vi "Add Property to Schema.vi"(4 "Typedef Name":string, 6 "Typedef?":bool, 8 "error in":errorcluster, 9 "JSON Schema Property in":string, 10 "Property Name":string, 11 "JSON Schema in":string) -> (0 "error out":errorcluster, 3 "JSON Schema out":string)   [LabVIEW 2023, in "JSON Schema Generator.lvlib"]
uses:
  JSON Schema Generator.lvlib
  <vilib>/JDP Science/JSONtext/Get all Object Items.vi
  <vilib>/JDP Science/JSONtext/Set Multiple Object Items.vi
  <vilib>/JDP Science/JSONtext/JSONtext.lvlib
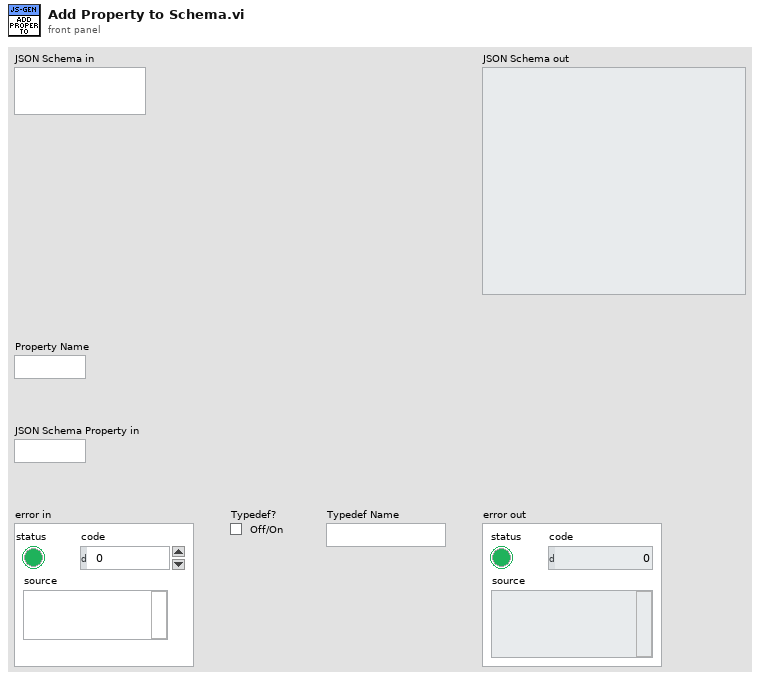
[diagram p1: front panel]
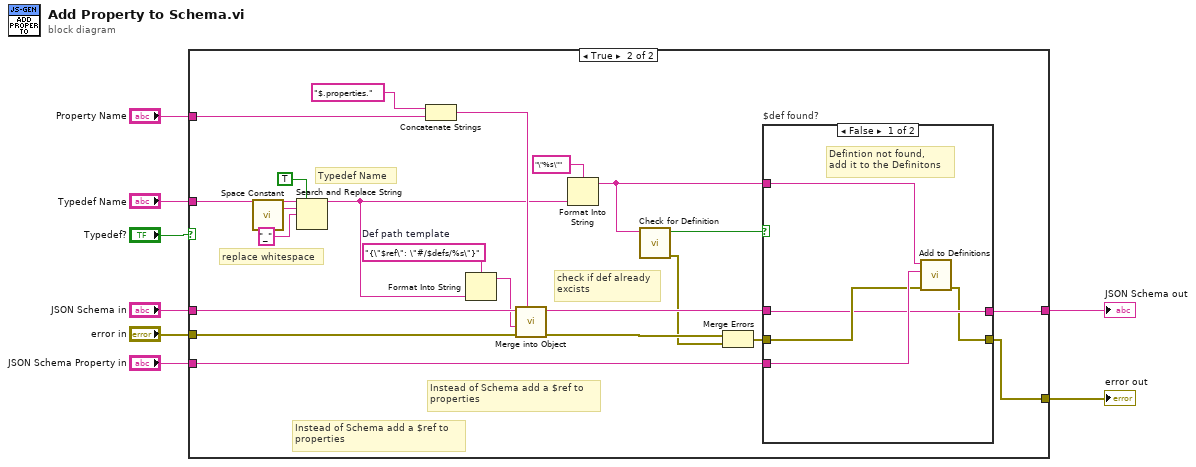
[diagram p0: block diagram]
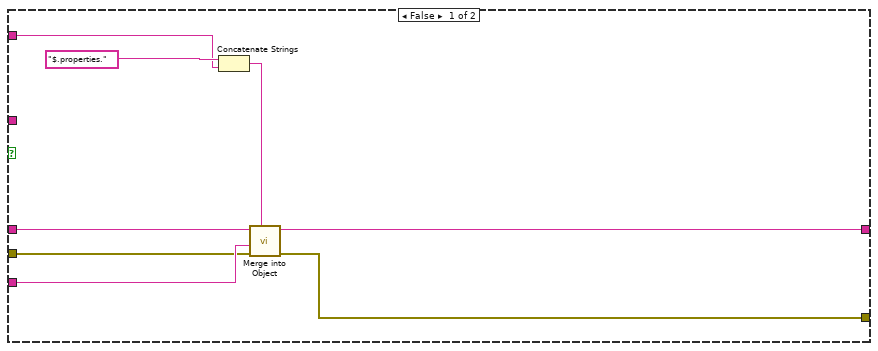
[diagram p2: hidden frame]
diagram:
  n1 = case shown="True" "Typedef?" {
    tunnel: "JSON Schema in" -> [w16 w37]
    tunnel: [w15 w18] -> w7
    tunnel: "Property Name" -> [w12 w33]
    tunnel: "JSON Schema Property in" -> [w11 w35]
    tunnel: "error in" -> [w10 w36]
    tunnel: [w9 w17] -> w3
    tunnel: "Typedef Name" -> [_ w22]
    frame False {
      n2 = Concatenate Strings("$.properties." ("$Path or Item Name"), w12) -> (w13:string)
      n3 = call <vilib>:"Merge into Object.vi"("$Path or Item Name"=w13, "error in (no error)"=w10, "JSON Object to Merge"=w11, "JSON"=w16) -> ("error out"=w9:errorcluster, "<JSON>"=w15:string)  [unwired: 5 in]
    }
    frame True {
      w29 = "{\"$ref\": \"#/$defs/%s\"}"  # Def path template
      # "Typedef Name"
      # "check if def already\nexcists"
      # "replace whitespace"
      # "Instead of Schema add a $ref to \nproperties"
      # "Instead of Schema add a $ref to \nproperties"
      n4 = call <vilib>:"Space Constant.vi"() -> ("String"=w27:string)
      n5 = Search and Replace String(replace all?=TRUE ("replace all? (F)"), input string=w22, search string=w27, replace string="_" ("replace string (\"\")")) -> (result string=w24:string)  [unwired: 4 in, 3 out]
      n6 = Concatenate Strings("$.properties." ("$Path or Item Name"), w33) -> (w34:string)
      n7 = Format Into String(format string=w29, w24) -> (resulting string=w23:string)  [unwired: 2 in, 1 out]
      n8 = call <vilib>:"Merge into Object.vi"("$Path or Item Name"=w34, "error in (no error)"=w36, "JSON Object to Merge"=w23, "JSON"=w37) -> ("error out"=w31:errorcluster, "<JSON>"=w32:string)  [unwired: 5 in]
      n9 = Format Into String(format string="\"%s\"", w24) -> (resulting string=w20:string)  [unwired: 2 in, 1 out]
      n10 = call "Check for Definition.vi"("Definition Name"=w20) -> ("error out"=w19:errorcluster, "Found?"=w21:bool)  [unwired: 9 in]
      n11 = Merge Errors(w31, w19) -> (w30:errorcluster)
      n12 = case "$def found?" shown="False" w21 {
        tunnel: [w41 w45] -> w18
        tunnel: [w40 w44] -> w17
        tunnel: w35 -> [w43 _]
        tunnel: w20 -> [w39 _]
        tunnel: w32 -> [w41 w45]
        tunnel: w30 -> [w42 w44]
        frame False {
          # "Defintion not found, \nadd it to the Definitons"
          n13 = call "Add to Definitions.vi"("error in (no error)"=w42, "Definition Schema"=w43, "Name"=w39) -> ("error out"=w40:errorcluster)  [unwired: 8 in]
        }
        frame True {
          # "Defintion  found"
        }
      }
    }
  }
  "error out" <- w3
  "JSON Schema out" <- w7
